vi "MultiScanDrift_dev.vi"() -> ()   [LabVIEW 2014]
uses:
  shared/CorrelImages (SubVI)Single.vi
  <userlib>/Nanonis Prog Interface V5/Nanonis Prog Interface.lvlib
panel:
  out "Number of Rows":u32
  in  "Lockin ON/OFF":bool
  in  "Multipass":bool=TRUE
  in  "Add":bool
  in  "end":sgl=1.0 format="%#_6p"
  in  "step":sgl=0.05 format="%#_6p"
  in  "start":sgl=-1.5 format="%#_6p"
  in  "create Range":bool
  in  "PLL ON/OFF":bool
  in  "ref bias":dbl=-0.0012 format="%#_6p"
  in  "ref setpoint":bool
  in  "DC On":bool=TRUE
  out "Y drift":i32
  out "X drift":i32
  out "DC active":bool
  in  "Drift correction Pixels":i32=128
  in  "Img Current":sgl=1e-10 format="%#_6p"
  in  "Img Bias (V) DC":sgl=1.0 format="%_2p"
  in  "Forward Speed":sgl=1.2e-09 format="%#_6p"
  in  "Backward Speed":sgl=8e-08 format="%#_6p"
  in  "Img Speed":sgl=4.5e-08 format="%#_6p"
  in  "Channel index (0-23)":u8(ring) items=["Current"=0, "Z (m)"=14]
  in  "Settling time (s)":dbl=0.7 format="%#_6p"
  in  "img bias":bool
  in  "img bias":dbl=-0.0012 format="%#_6p"
  in  "img delay (s)":u32=1
  out "tipLift":dbl format="%#_6p"
  in  "TipLiftList":i32(listbox)
  in  "Const Height":bool
  in  "CurrentList":i32(listbox)
  in  "BiasList":i32(listbox)=35
  out "Current":dbl=5e-11 format="%#_6p"
  out "Bias":dbl=0.02 format="%#_6p"
  # "Turn continuous scan off\n zero tiplift is '0'"
  # "Multipass Windows \nneeds to be open\n and OFF"
  # "5"
  # "10"
  # "15"
  # "20"
  # "25"
  # "30"
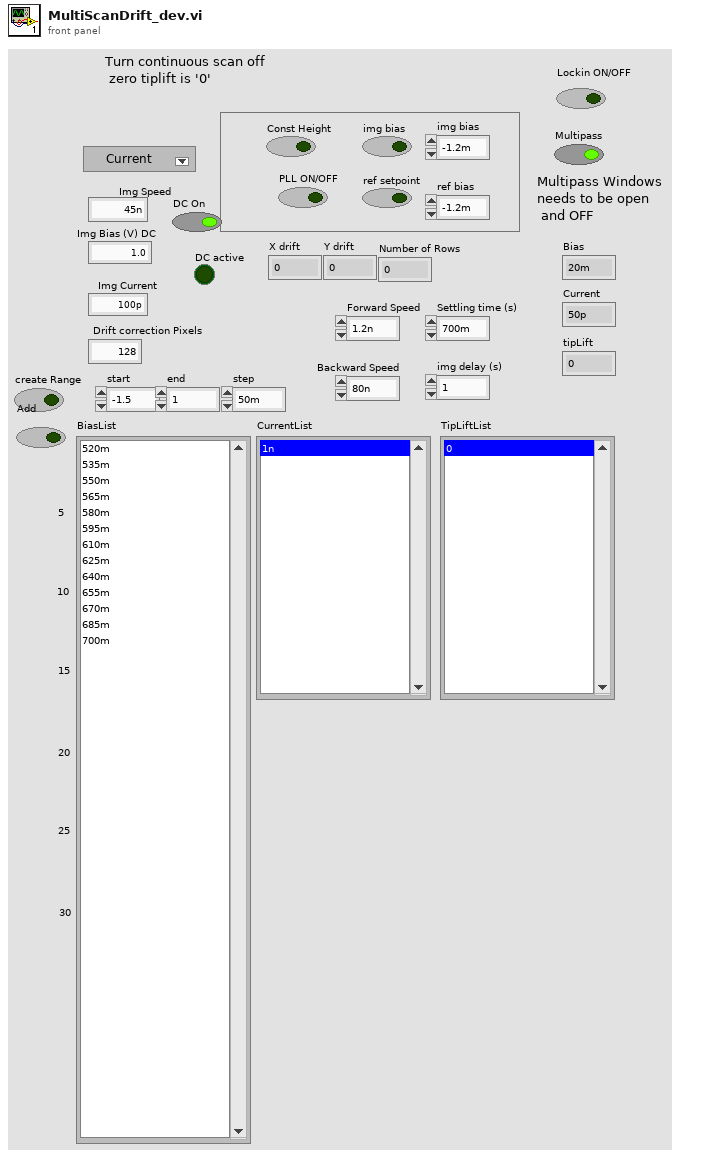
[diagram p1: front panel]
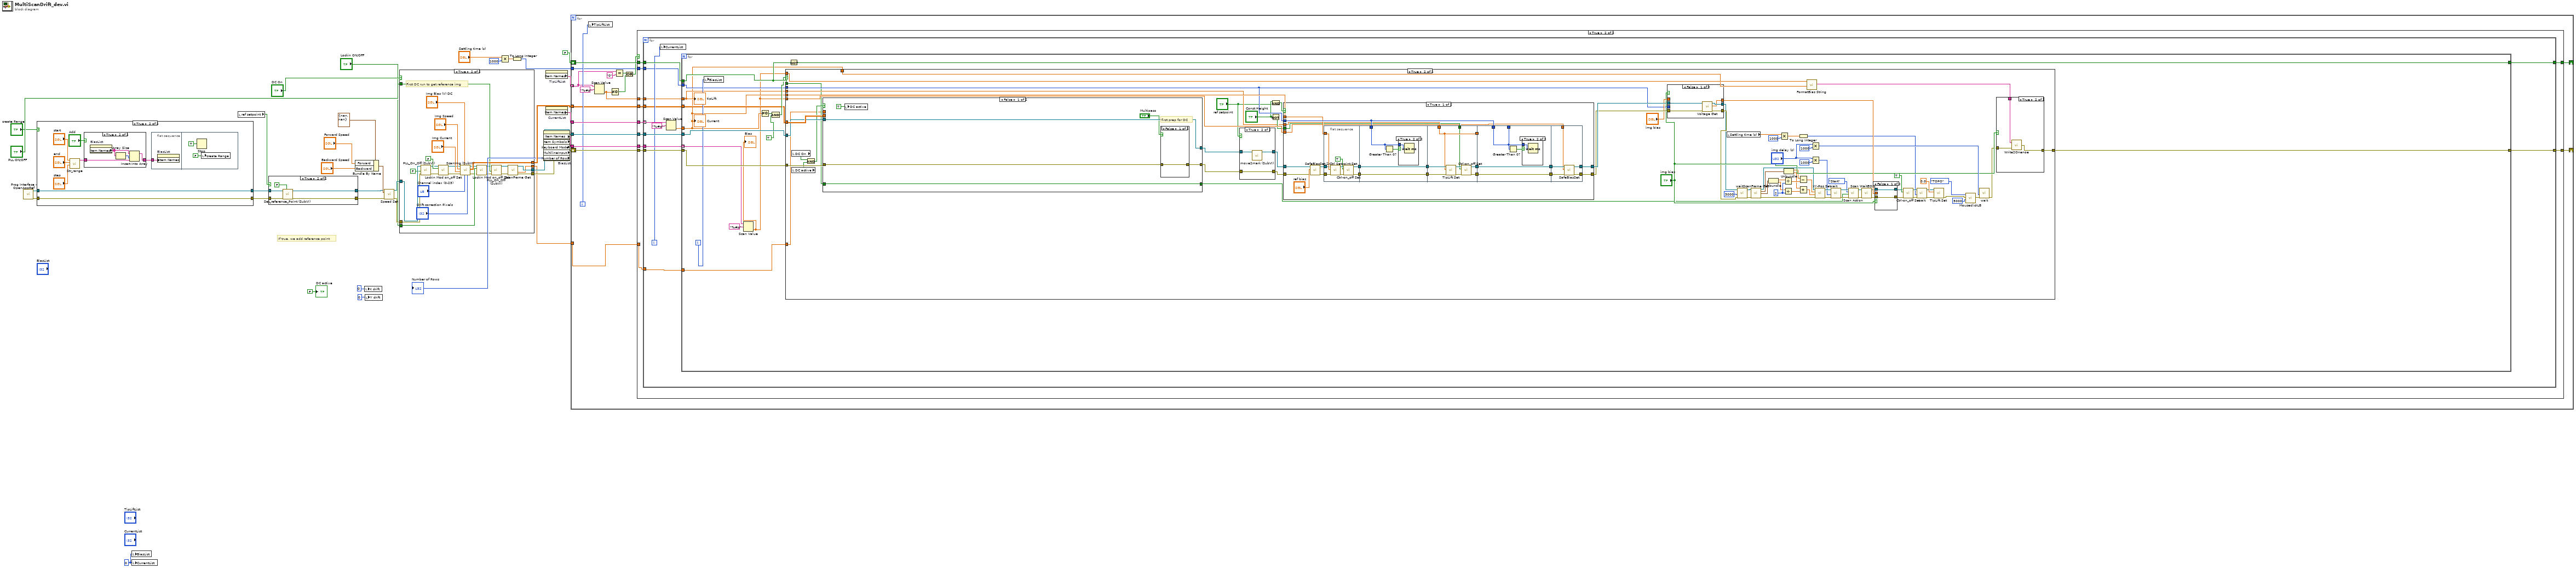
[diagram p0: block diagram]
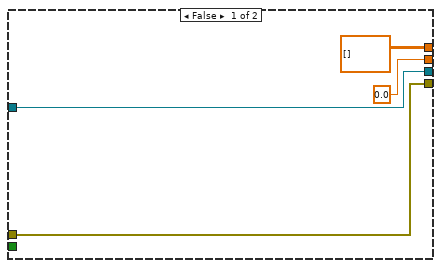
[diagram p5: hidden frame]
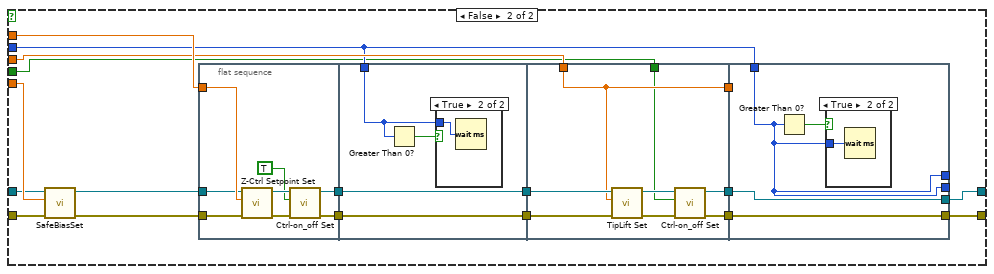
[diagram p11: hidden frame]
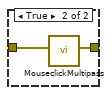
[diagram p15: hidden frame]
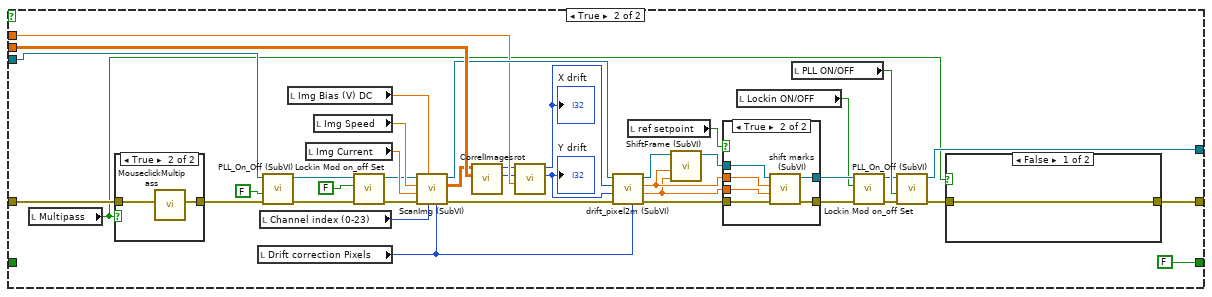
[diagram p16: hidden frame]
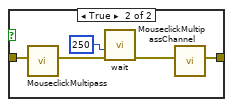
[diagram p18: hidden frame]
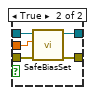
[diagram p20: hidden frame]
diagram:
  w34 = 0 ("BiasList")
  # "If true, we add reference point"
  n1 = call <userlib>:"Prog Interface - OpenAppRef.vi"() -> ("Error out"=w8:errorcluster, "Application reference"=w9:refnum<vi>)  [unwired: 6 in]
  n2 = case shown="True" "create Range" {
    tunnel: w9 -> [w36 w44]
    tunnel: [w36 w44] -> w4
    tunnel: w8 -> [w35 w43]
    tunnel: [w35 w43] -> w6
    frame False {
    }
    frame True {
      n3 = call "Str_range.vi"("step"="step", "end"="end", "start"="start") -> ("Item Names"=w37:string[])  [unwired: 8 in]
      n4 = case shown="True" "Add" {
        tunnel: [w48 w50] -> w38
        tunnel: w37 -> [w48 w49]
        frame False {
        }
        frame True {
          n5 = property on="BiasList" class="LstBox (strict)"() -> ("Item Names"=w51:string[])  [unwired: 2 in, 2 out]
          n6 = Array Size(array=w51) -> (size(s)=w52:i32)
          n7 = Insert Into Array(array=w51, index=w52, new element=w49) -> (w50:string[])
        }
      }
      n8 = flat-sequence {
        tunnel: w38 -> [w45]
        frame #0 {
          n9 = property on="BiasList" class="LstBox (strict)"("Item Names"=w45) -> ()  [unwired: 2 in, 2 out]
        }
        frame #1 {
          n10 = Stop(stop? (T)=TRUE) -> ()
          n11 = local write "create Range"(FALSE ("Range")) -> ()
        }
      }
    }
  }
  n12 = local write "BiasList"(w34) -> ()
  n13 = local write "CurrentList"(w34) -> ()
  n14 = local read "ref setpoint"() -> (w7:bool)
  n15 = case shown="True" w7 {
    tunnel: w6 -> [w54 w58]
    tunnel: [w54 w57] -> w5
    tunnel: w4 -> [w53 w56]
    tunnel: [w53 w55] -> w3
    frame False {
    }
    frame True {
      n16 = call "Set_reference_Point (SubVI).vi"("Part of multigrid"=FALSE, "error in (no error)"=w58, "Application in"=w56) -> ("error out"=w57:errorcluster, "Application out"=w55:refnum<vi>)  [unwired: 7 in]
    }
  }
  n17 = Bundle By Name(cluster=cluster{"Forward":sgl, "Backward":sgl} {"Forward"=nan, "Backward"=nan} ("Speed (m/s)"), "Forward"="Forward Speed", "Backward"="Backward Speed") -> (w20:cluster{"Forward":sgl, "Backward":sgl})
  n18 = local write "X drift"(0 ("X drift")) -> ()
  n19 = local write "Y drift"(0 ("Y drift")) -> ()
  n20 = call <userlib>:"Speed Set.vi"("Application ref in"=w3, "Speed (m/s)"=w20, "error in (no error)"=w5) -> ("Application ref out"=w18:refnum<vi>, "error out"=w17:errorcluster)  [unwired: 11 in]
  n21 = case shown="True" "DC On" {
    tunnel: [w62 w77] -> w22
    tunnel: [w61 w76] -> w21
    tunnel: [dbl[][] [] ("Img") w84] -> w19
    tunnel: w18 -> [w62 w83]
    tunnel: w17 -> [w61 w82]
    tunnel: [sgl 0.0 ("Angle (deg)") w75] -> w12
    tunnel: "PLL ON/OFF" -> [_ w74]
    tunnel: "Lockin ON/OFF" -> [_ w68]
    frame False {
    }
    frame True {
      # "First DC run to get reference img"
      n22 = call "PLL_On_Off (SubVI).vi"("error in (no error)"=w82, "Output ON/OFF (F=OFF)"=FALSE, "Application in"=w83) -> ("error out"=w71:errorcluster, "Application out"=w72:refnum<vi>)  [unwired: 7 in]
      n23 = call <userlib>:"Lockin Mod on_off Set.vi"("Error in (no error)"=w71, "Lockin ON/OFF"=FALSE, "Application ref in"=w72) -> ("Error out"=w70:errorcluster, "Application ref out"=w69:refnum<vi>)  [unwired: 7 in]
      n24 = call "ScanImg (SubVI).vi"("pixel"="Drift correction Pixels", "Channel index (0-23)"="Channel index (0-23)", "Bias (V)"="Img Bias (V) DC", "error in (no error)"=w70, "Current"="Img Current", "Img Speed"="Img Speed", "Application in"=w69) -> ("error out"=w65:errorcluster, "Img"=w84:dbl[][], "Application out"=w67:refnum<vi>)  [unwired: 2 in]
      n25 = call <userlib>:"Lockin Mod on_off Set.vi"("Error in (no error)"=w65, "Lockin ON/OFF"=w68, "Application ref in"=w67) -> ("Error out"=w64:errorcluster, "Application ref out"=w66:refnum<vi>)  [unwired: 7 in]
      n26 = call "PLL_On_Off (SubVI).vi"("error in (no error)"=w64, "Output ON/OFF (F=OFF)"=w74, "Application in"=w66) -> ("error out"=w78:errorcluster, "Application out"=w79:refnum<vi>)  [unwired: 7 in]
      n27 = call <userlib>:"ScanFrame Get.vi"("Application ref in"=w79, "error in (no error)"=w78) -> ("Application ref out"=w77:refnum<vi>, "Angle (deg)"=w75:sgl, "error out"=w76:errorcluster)  [unwired: 9 in, 2 out]
    }
  }
  n28 = Multiply(x="Settling time (s)", y=u32 1000) -> (x*y=w30:dbl)
  n29 = To Long Integer(number=w30) -> (32bit integer=w31:i32)
  n30 = property on="BiasList" class="LstBox (strict)" props=["Item Names", "Item Symbols", "Keyboard Mode", "MultilineInput", "Number of Rows"]() -> ("Item Names"=w28:string[], "Number of Rows"=→"Number of Rows":u32)  [unwired: 2 in, 5 out]
  n31 = property on="TipLiftList" class="LstBox (strict)"() -> ("Item Names"=w26:string[])  [unwired: 2 in, 2 out]
  n32 = property on="CurrentList" class="LstBox (strict)"() -> ("Item Names"=w27:string[])  [unwired: 2 in, 2 out]
  n33 = for {
    tunnel: w28 -> [w105]
    tunnel: w27 -> [w104]
    tunnel: w22 -> [w103]
    tunnel: w26 -> [w99] mode=indexing
    shift-right: [w93] -> _
    shift-left: FALSE ("Direction: up/down (T=up)") -> [w106]
    tunnel: w31 -> [w92]
    tunnel: w19 -> [w91]
    tunnel: w12 -> [w90]
    shift-right: [w89] -> _
    shift-left: w21 -> [w102]
    i -> [w100]
    n34 = local write "TipLiftList"(w100) -> ()
    n35 = Scan Value(string=w99, format string="%#p") -> (value=w98:dbl)  [unwired: 1 in, 1 out]
    n36 = Not Equal To 0?(x=w98) -> (x != 0?=w97:bool)
    n37 = Equal?(x=w99, y="0") -> (x = y?=w94:bool)
    n38 = Or(x=w94, y=w97) -> (x .or. y?=w96:bool)
    n39 = case shown="True" w96 {
      tunnel: w106 -> [w108 w119]
      tunnel: w105 -> [_ w118]
      tunnel: w104 -> [_ w117]
      tunnel: w103 -> [_ w116]
      tunnel: w102 -> [w107 w115]
      tunnel: w98 -> [_ w114]
      tunnel: [w108 w113] -> w93
      tunnel: w92 -> [_ w112]
      tunnel: w91 -> [_ w111]
      tunnel: w90 -> [_ w110]
      tunnel: [w107 w109] -> w89
      frame False {
      }
      frame True {
        n40 = for {
          tunnel: w119 -> [w133]
          tunnel: w116 -> [w132]
          tunnel: w115 -> [w131]
          tunnel: w118 -> [w130]
          tunnel: w117 -> [w128] mode=indexing
          tunnel: w114 -> [w125]
          tunnel: [w124] -> w113
          tunnel: w112 -> [w123]
          tunnel: w111 -> [w122]
          tunnel: w110 -> [w121]
          tunnel: [w120] -> w109
          i -> [w126]
          n41 = local write "CurrentList"(w126) -> ()
          n42 = Scan Value(string=w128, format string="%#p") -> (value=w127:dbl)  [unwired: 1 in, 1 out]
          n43 = for {
            tunnel: w130 -> [w136] mode=indexing
            tunnel: w132 -> [w148]
            tunnel: w131 -> [w147]
            tunnel: w127 -> [w139]
            tunnel: w125 -> [w143]
            tunnel: w133 -> [w150]
            tunnel: [w149] -> w124
            tunnel: w123 -> [w142]
            tunnel: w122 -> [w141]
            tunnel: w121 -> [w140]
            tunnel: [w138] -> w120
            i -> [w144]
            n44 = local write "BiasList"(w144) -> ()
            n45 = Scan Value(string=w136, format string="%#p") -> (value=w137:dbl)  [unwired: 1 in, 1 out]
            "Bias" <- w137
            n46 = Not Equal To 0?(x=w139) -> (x != 0?=w146:bool)
            n47 = Compound Arithmetic op=AND(w146, TRUE) -> (w145:bool)
            n48 = case shown="True" w145 {
              tunnel: w150 -> [_ w203]
              tunnel: w137 -> [_ w229]
              tunnel: w148 -> [_ w208]
              tunnel: w147 -> [w151 w207]
              tunnel: w139 -> [_ w230]
              tunnel: w143 -> [_ w226]
              tunnel: w142 -> [_ w210]
              tunnel: w141 -> [_ w209]
              tunnel: w140 -> [_ w202]
              tunnel: w137 -> [_ w201]
              tunnel: w139 -> [_ w200]
              tunnel: [w151 w196] -> w138
              frame False {
              }
              frame True {
                w182 = 2
                n49 = local read "DC On"() -> (w205:bool)
                n50 = local read "DC active"() -> (w206:bool)
                n51 = And(x=w205, y=w206) -> (x .and. y?=w204:bool)
                n52 = case shown="False" w204 {
                  tunnel: w209 -> [_ w384]
                  tunnel: w208 -> [w341 w376]
                  tunnel: w207 -> [w337 w365]
                  tunnel: [w336 w361] -> w162
                  tunnel: [w341 w375] -> w163
                  tunnel: [w339 FALSE ("Direction: up/down (T=up)")] -> w167
                  tunnel: w203 -> [w339 _]
                  tunnel: w202 -> [_ w371]
                  frame False {
                    # "first prep for DC"
                    n53 = local write "DC active"(TRUE ("DC active")) -> ()
                    n54 = case shown="False" "Multipass" {
                      tunnel: w337 -> [w342 w344]
                      tunnel: [w342 w343] -> w336
                      frame False {
                      }
                      frame True {
                        n55 = call "MouseclickMultipass.vi"("error in (no error)"=w344) -> ("error out"=w343:errorcluster)  [unwired: 10 in]
                      }
                    }
                  }
                  frame True {
                    n56 = local read "Multipass"() -> (w360:bool)
                    n57 = case shown="True" w360 {
                      tunnel: w365 -> [w399 w401]
                      tunnel: [w399 w400] -> w364
                      frame False {
                      }
                      frame True {
                        n58 = call "MouseclickMultipass.vi"("error in (no error)"=w401) -> ("error out"=w400:errorcluster)  [unwired: 10 in]
                      }
                    }
                    n59 = local read "Drift correction Pixels"() -> (w373:i32)
                    n60 = local read "Channel index (0-23)"() -> (w379:u8)
                    n61 = call "PLL_On_Off (SubVI).vi"("error in (no error)"=w364, "Output ON/OFF (F=OFF)"=FALSE, "Application in"=w376) -> ("error out"=w354:errorcluster, "Application out"=w352:refnum<vi>)  [unwired: 7 in]
                    n62 = local read "Img Bias (V) DC"() -> (w380:sgl)
                    n63 = local read "Img Current"() -> (w381:sgl)
                    n64 = local read "Img Speed"() -> (w382:sgl)
                    n65 = call <userlib>:"Lockin Mod on_off Set.vi"("Error in (no error)"=w354, "Lockin ON/OFF"=FALSE, "Application ref in"=w352) -> ("Error out"=w353:errorcluster, "Application ref out"=w351:refnum<vi>)  [unwired: 7 in]
                    n66 = call "ScanImg (SubVI).vi"("pixel"=w373, "Channel index (0-23)"=w379, "Bias (V)"=w380, "error in (no error)"=w353, "Current"=w381, "Img Speed"=w382, "Application in"=w351) -> ("error out"=w363:errorcluster, "Img"=w383:dbl[][], "Application out"=w377:refnum<vi>)  [unwired: 2 in]
                    n67 = call-poly "CorrelImages.vi"("Ref Array"=w384, "New Image"=w383) -> ("Y drift"=w368:i32, "X drift"=w370:i32)  [unwired: 6 in, 2 out]
                    n68 = call "rot.vi"("angle"=w371, "y"=w368, "x"=w370) -> ("y'"=w367:i32, "x'"=w369:i32)  [unwired: 7 in]
                    "X drift" <- w369
                    "Y drift" <- w367
                    n69 = call "drift_pixel2m (SubVI).vi"("Application in"=w377, "X drift"=w369, "Y drift"=w367, "error in"=w363, "Drift correction Pixels"=w373) -> ("Application out"=w378:refnum<vi>, "x drift"=w358:sgl, "y drift"=w357:sgl, "error out"=w356:errorcluster)  [unwired: 1 in]
                    n70 = local read "ref setpoint"() -> (w359:bool)
                    n71 = call "ShiftFrame (SubVI).vi"("Y shift"=w357, "X shift"=w358, "Application in"=w378) -> ("Application out"=w355:refnum<vi>)  [unwired: 8 in]
                    n72 = case shown="True" w359 {
                      tunnel: w358 -> [_ w392]
                      tunnel: w357 -> [_ w391]
                      tunnel: w356 -> [w385 w390]
                      tunnel: [w385 w389] -> w347
                      tunnel: w355 -> [w386 w388]
                      tunnel: [w386 w387] -> w346
                      frame False {
                      }
                      frame True {
                        n73 = call "shift marks (SubVI).vi"("error in (no error)"=w390, "y"=w391, "x"=w392, "Application in"=w388) -> ("error out"=w389:errorcluster, "Application out"=w387:refnum<vi>)  [unwired: 6 in]
                      }
                    }
                    n74 = local read "Lockin ON/OFF"() -> (w345:bool)
                    n75 = local read "PLL ON/OFF"() -> (w366:bool)
                    n76 = call <userlib>:"Lockin Mod on_off Set.vi"("Error in (no error)"=w347, "Lockin ON/OFF"=w345, "Application ref in"=w346) -> ("Error out"=w348:errorcluster, "Application ref out"=w349:refnum<vi>)  [unwired: 7 in]
                    n77 = call "PLL_On_Off (SubVI).vi"("error in (no error)"=w348, "Output ON/OFF (F=OFF)"=w366, "Application in"=w349) -> ("error out"=w362:errorcluster, "Application out"=w375:refnum<vi>)  [unwired: 7 in]
                    n78 = case shown="False" w360 {
                      tunnel: w362 -> [w393 w398]
                      tunnel: [w393 w397] -> w361
                      frame False {
                      }
                      frame True {
                        n79 = call "MouseclickMultipass.vi"("error in (no error)"=w398) -> ("error out"=w396:errorcluster)  [unwired: 10 in]
                        n80 = call "wait.vi"("error in"=w396, "milliseconds to wait"=u32 250) -> ("error out"=w395:errorcluster)  [unwired: 8 in, 1 out]
                        n81 = call "MouseclickMultipassChannel.vi"("error in (no error)"=w395) -> ("error out"=w397:errorcluster)  [unwired: 10 in]
                      }
                    }
                  }
                }
                n82 = case shown="True" "ref setpoint" {
                  tunnel: w163 -> [w232 w235]
                  tunnel: w162 -> [w231 w234]
                  tunnel: [w231 w234] -> w160
                  tunnel: [w232 w233] -> w161
                  frame False {
                  }
                  frame True {
                    n83 = call "move2mark (SubVI).vi"("Application in"=w235) -> ("Application out"=w233:refnum<vi>)  [unwired: 10 in]
                  }
                }
                n84 = Not(x="Const Height") -> (.not. x?=w228:bool)
                n85 = And(x="Const Height", y="ref setpoint") -> (x .and. y?=w194:bool)
                n86 = case shown="True" w194 {
                  tunnel: w230 -> [w243 w295]
                  tunnel: w229 -> [w238 w305]
                  tunnel: w228 -> [w239 w290]
                  tunnel: w226 -> [w240 w292]
                  tunnel: [w237 w289] -> w223
                  tunnel: [w236 w288] -> w222
                  tunnel: w210 -> [w244 w291]
                  tunnel: w160 -> [w254 w304]
                  tunnel: w161 -> [w255 w303]
                  frame True {
                    n87 = call "SafeBiasSet.vi"("Application ref in"=w255, "Bias (V)"="ref bias", "error in (no error)"=w254) -> ("Application ref out"=w242:refnum<vi>, "Error out"=w241:errorcluster)  [unwired: 6 in]
                    n88 = flat-sequence {
                      tunnel: [w263] -> w253
                      tunnel: [w260] -> w252
                      tunnel: w243 -> [w259]
                      tunnel: w242 -> [w258]
                      tunnel: w241 -> [w257]
                      tunnel: w253 -> [w268]
                      tunnel: [w268] -> w251
                      tunnel: w244 -> [w266]
                      tunnel: [w265] -> w250
                      tunnel: w252 -> [w265]
                      tunnel: w251 -> [w277]
                      tunnel: [w275] -> w249
                      tunnel: [w271] -> w248
                      tunnel: w250 -> [w274]
                      tunnel: [w272] -> w247
                      tunnel: w240 -> [w271]
                      tunnel: w239 -> [w270]
                      tunnel: w249 -> [w281]
                      tunnel: [w278] -> _
                      tunnel: w248 -> [_]
                      tunnel: [w281] -> w246
                      tunnel: [w279] -> w245
                      tunnel: w247 -> [w279]
                      tunnel: w244 -> [w278]
                      tunnel: [w286] -> w237
                      tunnel: w246 -> [w287]
                      tunnel: w245 -> [w285]
                      tunnel: [w284] -> w236
                      tunnel: w238 -> [w283]
                      frame #0 {
                        n89 = call <userlib>:"Z-Ctrl Setpoint Set.vi"("error in (no error)"=w257, "Z Controller setpoint"=w259, "Application ref in"=w258) -> ("error out"=w261:errorcluster, "Application ref out"=w264:refnum<vi>)  [unwired: 7 in]
                        n90 = call <userlib>:"Ctrl-on_off Set.vi"("error in (no error)"=w261, "Z Controller ON/OFF"=TRUE, "Application ref in"=w264) -> ("error out"=w260:errorcluster, "Application ref out"=w263:refnum<vi>)  [unwired: 7 in]
                      }
                      frame #1 {
                        n91 = Greater Than 0?(x=w266) -> (x > 0?=w267:bool)
                        n92 = case shown="True" w267 {
                          tunnel: w266 -> [_ w269]
                          frame False {
                          }
                          frame True {
                            n93 = Wait (ms)(milliseconds to wait=w269) -> ()  [unwired: 1 out]
                          }
                        }
                      }
                      frame #2 {
                        n94 = call <userlib>:"TipLift Set.vi"("error in (no error)"=w274, "TipLift (m)"=w271, "Application ref in"=w277) -> ("error out"=w273:errorcluster, "Application ref out"=w276:refnum<vi>)  [unwired: 7 in]
                        n95 = call <userlib>:"Ctrl-on_off Set.vi"("error in (no error)"=w273, "Z Controller ON/OFF"=w270, "Application ref in"=w276) -> ("error out"=w272:errorcluster, "Application ref out"=w275:refnum<vi>)  [unwired: 7 in]
                      }
                      frame #3 {
                        n96 = Greater Than 0?(x=w278) -> (x > 0?=w280:bool)
                        n97 = case shown="True" w280 {
                          tunnel: w278 -> [_ w282]
                          frame False {
                          }
                          frame True {
                            n98 = Wait (ms)(milliseconds to wait=w282) -> ()  [unwired: 1 out]
                          }
                        }
                      }
                      frame #4 {
                        n99 = call "SafeBiasSet.vi"("Application ref in"=w287, "Bias (V)"=w283, "error in (no error)"=w285) -> ("Application ref out"=w286:refnum<vi>, "Error out"=w284:errorcluster)  [unwired: 6 in]
                      }
                    }
                  }
                  frame False {
                    n100 = call "SafeBiasSet.vi"("Application ref in"=w303, "Bias (V)"=w305, "error in (no error)"=w304) -> ("Application ref out"=w294:refnum<vi>, "Error out"=w293:errorcluster)  [unwired: 6 in]
                    n101 = flat-sequence {
                      tunnel: [w312] -> w302
                      tunnel: [w309] -> w301
                      tunnel: w295 -> [w308]
                      tunnel: w294 -> [w307]
                      tunnel: w293 -> [w306]
                      tunnel: w302 -> [w317]
                      tunnel: [w317] -> w300
                      tunnel: w291 -> [w315]
                      tunnel: [w314] -> w299
                      tunnel: w301 -> [w314]
                      tunnel: w300 -> [w326]
                      tunnel: [w324] -> w298
                      tunnel: [w320] -> w297
                      tunnel: w299 -> [w323]
                      tunnel: [w321] -> w296
                      tunnel: w292 -> [w320]
                      tunnel: w290 -> [w319]
                      tunnel: w291 -> [w329]
                      tunnel: [w329] -> _
                      tunnel: w296 -> [w327]
                      tunnel: w297 -> [_]
                      tunnel: [w329] -> _
                      tunnel: w298 -> [w328]
                      tunnel: [w328] -> w289
                      tunnel: [w327] -> w288
                      frame #0 {
                        n102 = call <userlib>:"Z-Ctrl Setpoint Set.vi"("error in (no error)"=w306, "Z Controller setpoint"=w308, "Application ref in"=w307) -> ("error out"=w310:errorcluster, "Application ref out"=w313:refnum<vi>)  [unwired: 7 in]
                        n103 = call <userlib>:"Ctrl-on_off Set.vi"("error in (no error)"=w310, "Z Controller ON/OFF"=TRUE, "Application ref in"=w313) -> ("error out"=w309:errorcluster, "Application ref out"=w312:refnum<vi>)  [unwired: 7 in]
                      }
                      frame #1 {
                        n104 = Greater Than 0?(x=w315) -> (x > 0?=w316:bool)
                        n105 = case shown="True" w316 {
                          tunnel: w315 -> [_ w318]
                          frame False {
                          }
                          frame True {
                            n106 = Wait (ms)(milliseconds to wait=w318) -> ()  [unwired: 1 out]
                          }
                        }
                      }
                      frame #2 {
                        n107 = call <userlib>:"TipLift Set.vi"("error in (no error)"=w323, "TipLift (m)"=w320, "Application ref in"=w326) -> ("error out"=w322:errorcluster, "Application ref out"=w325:refnum<vi>)  [unwired: 7 in]
                        n108 = call <userlib>:"Ctrl-on_off Set.vi"("error in (no error)"=w322, "Z Controller ON/OFF"=w319, "Application ref in"=w325) -> ("error out"=w321:errorcluster, "Application ref out"=w324:refnum<vi>)  [unwired: 7 in]
                      }
                      frame #3 {
                        n109 = Greater Than 0?(x=w329) -> (x > 0?=w330:bool)
                        n110 = case shown="True" w330 {
                          tunnel: w329 -> [_ w331]
                          frame False {
                          }
                          frame True {
                            n111 = Wait (ms)(milliseconds to wait=w331) -> ()  [unwired: 1 out]
                          }
                        }
                      }
                    }
                  }
                }
                n112 = case shown="False" "img bias" {
                  tunnel: w223 -> [w413 w420]
                  tunnel: [w412 w416] -> w165
                  tunnel: w222 -> [w409 w423]
                  tunnel: [w410 w417] -> w166
                  tunnel: "img bias" -> [_ w418]
                  tunnel: [w411 w424] -> w220
                  tunnel: w210 -> [_ w419]
                  frame False {
                    n113 = call <userlib>:"Voltage Get.vi"("error in (no error)"=w409, "Application ref in"=w413) -> ("error out"=w410:errorcluster, "Bias (V)"=w411:sgl, "Application ref out"=w412:refnum<vi>)  [unwired: 7 in]
                  }
                  frame True {
                    n114 = call "wait.vi"("error in"=w423, "milliseconds to wait"=w419, "application reference in"=w420) -> ("error out"=w422:errorcluster, "application reference out"=w421:refnum<vi>)  [unwired: 7 in]
                    n115 = call <userlib>:"Voltage Get.vi"("error in (no error)"=w422, "Application ref in"=w421) -> ("error out"=w414:errorcluster, "Bias (V)"=w424:sgl, "Application ref out"=w415:refnum<vi>)  [unwired: 7 in]
                    n116 = call "SafeBiasSet.vi"("Application ref in"=w415, "Bias (V)"=w418, "error in (no error)"=w414) -> ("Application ref out"=w416:refnum<vi>, "Error out"=w417:errorcluster)  [unwired: 6 in]
                  }
                }
                n117 = local read "Settling time (s)"() -> (w153:dbl)
                n118 = call "wait.vi"("error in"=w166, "milliseconds to wait"=u32 3000 ("y"), "application reference in"=w165) -> ("error out"=w174:errorcluster, "application reference out"=w173:refnum<vi>)  [unwired: 7 in]
                n119 = call <userlib>:"ScanFrame Get.vi"("Application ref in"=w173, "error in (no error)"=w174) -> ("Application ref out"=w193:refnum<vi>, "Center coordinates (m)"=w177:cluster{"Xc":sgl, "Yc":sgl}, "Size (m)"=w178:cluster{"Width":sgl, "Height":sgl}, "error out"=w192:errorcluster)  [unwired: 9 in, 1 out]
                n120 = Unbundle(w178) -> ("Width"=w180:sgl, "Height"=w181:sgl)
                n121 = Multiply(x=w153, y=u32 1000) -> (x*y=w154:dbl)
                n122 = Divide(x=w180, y=w182) -> (x/y=w184:sgl)
                n123 = Divide(x=w181, y=w182) -> (x/y=w183:sgl)
                n124 = Unbundle(w177) -> ("Xc"=w185:sgl, "Yc"=w179:sgl)
                n125 = To Long Integer(number=w154) -> (32bit integer=w152:i32)
                n126 = Subtract(x=w185, y=w184) -> (x-y=w186:sgl)
                n127 = Add(x=w179, y=w183) -> (x+y=w187:sgl)
                n128 = call "FormatBias String.vi"("current"=w200, "bias"=w201) -> ("resulting string"=w197:string)  [unwired: 9 in]
                n129 = Multiply(x="img delay (s)", y=u32 1000) -> (x*y=w212:u32)
                n130 = Multiply(x="img delay (s)", y=u32 1000) -> (x*y=w189:u32)
                n131 = call <userlib>:"XY-Pos Set.vi"("error in (no error)"=w192, "Y (m)"=w187, "X (m)"=w186, "Application ref in"=w193) -> ("error out"=w191:errorcluster, "Application ref out"=w190:refnum<vi>)  [unwired: 4 in]
                n132 = call "wait.vi"("error in"=w191, "milliseconds to wait"=w189, "application reference in"=w190) -> ("error out"=w171:errorcluster, "application reference out"=w172:refnum<vi>)  [unwired: 7 in]
                n133 = call <userlib>:"Scan Action.vi"("error in (no error)"=w171, "Direction: up/down (T=up)"=w167, "Scan action (Start)"=enum16{"Start", "Stop", "Pause", "Resume"}."Start", "Application ref in"=w172) -> ("error out"=w169:errorcluster, "Application ref out"=w170:refnum<vi>)  [unwired: 5 in]
                n134 = call <userlib>:"Scan WaitEOS.vi"("error in (no error)"=w169, "Application ref in"=w170) -> ("error out"=w218:errorcluster, "Application ref out"=w219:refnum<vi>)  [unwired: 5 in, 2 out]
                n135 = case shown="False" "img bias" {
                  tunnel: w219 -> [w403 w404]
                  tunnel: [w403 w407] -> w217
                  tunnel: [w402 w408] -> w216
                  tunnel: w218 -> [w402 w406]
                  tunnel: w220 -> [_ w405]
                  frame False {
                  }
                  frame True {
                    n136 = call "SafeBiasSet.vi"("Application ref in"=w404, "Bias (V)"=w405, "error in (no error)"=w406) -> ("Application ref out"=w407:refnum<vi>, "Error out"=w408:errorcluster)  [unwired: 6 in]
                  }
                }
                n137 = call <userlib>:"Ctrl-on_off Set.vi"("error in (no error)"=w216, "Z Controller ON/OFF"=TRUE, "Application ref in"=w217) -> ("error out"=w159:errorcluster, "Application ref out"=w157:refnum<vi>)  [unwired: 7 in]
                n138 = call "wait.vi"("error in"=w159, "milliseconds to wait"=w152, "application reference in"=w157) -> ("error out"=w158:errorcluster, "application reference out"=w156:refnum<vi>)  [unwired: 7 in]
                n139 = call <userlib>:"TipLift Set.vi"("error in (no error)"=w158, "TipLift (m)"=sgl 0.0, "Application ref in"=w156) -> ("error out"=w225:errorcluster)  [unwired: 7 in, 1 out]
                n140 = call "MouseclickLB.vi"("nMilliseconds"=5000, "error in (no error)"=w225, "Click"=enum16{"Header", "TOPO", "STS", "GRID"}."TOPO") -> ("error out"=w211:errorcluster)  [unwired: 8 in]
                n141 = call "wait.vi"("error in"=w211, "milliseconds to wait"=w212) -> ("error out"=w198:errorcluster)  [unwired: 8 in, 1 out]
                n142 = case shown="True" "img bias" {
                  tunnel: w198 -> [w332 w335]
                  tunnel: w197 -> [_ w334]
                  tunnel: [w332 w333] -> w196
                  frame False {
                  }
                  frame True {
                    n143 = call "Write2Onenoe.vi"("error in (no error)"=w335, "strSendText"=w334) -> ("error out"=w333:errorcluster)
                  }
                }
              }
            }
            n144 = Not(x=w150) -> (.not. x?=w149:bool)
            "Current" <- w139
            "tipLift" <- w143
          }
        }
      }
    }
  }
  "DC active" <- FALSE ("DC active")
